vi "connectpython.vi"() -> ()   [LabVIEW 2019]
uses:
  <vilib>/Platform/TimedLoop/XDataNode/timing_clust.ctl
  <vilib>/Platform/TimedLoop/XDataNode/nitl_modes.ctl
  <vilib>/Platform/TimedLoop/XDataNode/wakeup.ctl
  <vilib>/platform/TimedLoop/XDataNode/XDataNode.xnode
  <vilib>/Platform/TimedLoop/XDataNode/XDNodeRunTimeDep.lvlib
panel:
  out "Waveform Chart":dbl(graph)
  out "data out":string
  out "xd":dbl
  out "yd":dbl
  out "phi":dbl
  out "error out":errorcluster
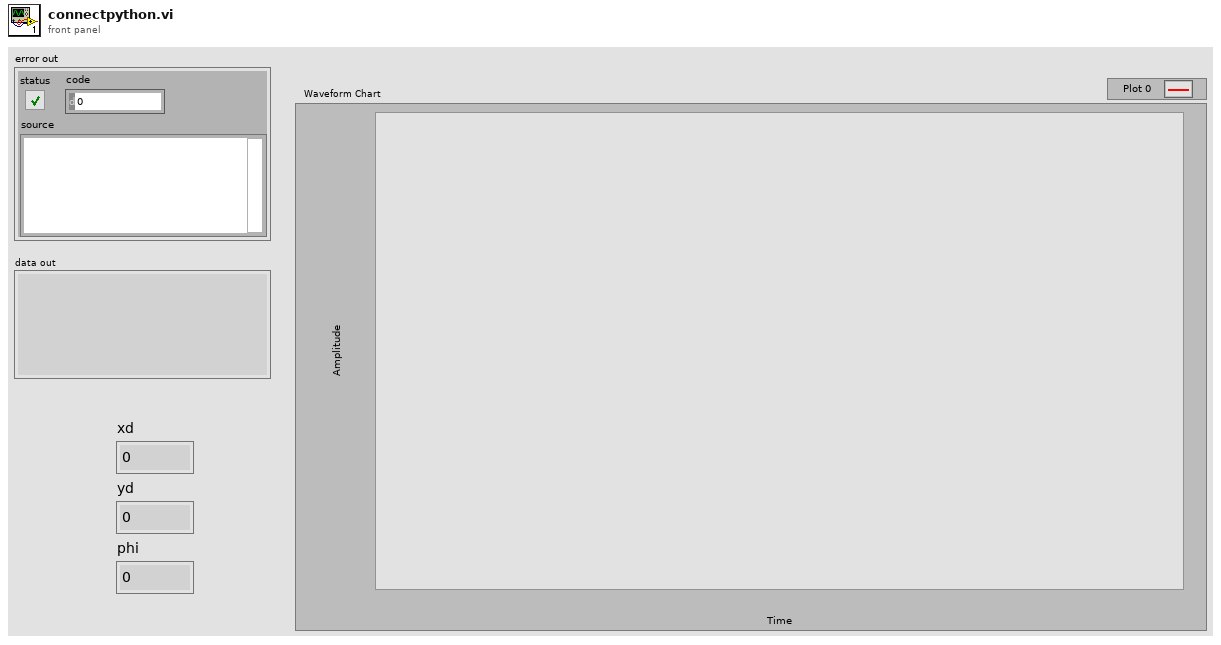
[diagram p1: front panel]
types:
  T1 = typedef "XDNodeRunTimeDep.lvlib/timing_clust.ctl" = cluster{"Expected End [f-1]":u64, "Actual End [f-1]":u64, "Finished Late? [f-1]":bool, "Expected End [i-1]":u64, "Actual End [i-1]":u64, "Finished Late? [i-1]":bool, "Expected Start [i]":u64, "Actual Start [i]":u64, "Expected Start [f]":u64, "Actual Start [f]":u64, "Source Name":string, "Structure Name":string, "Period":i64, "Deadline":i64, "Offset":i64, "Start":i64, "Priority":i32, "Timeout":i32, "Mode":T2, "Wakeup Reason":T3, "Error":errorcluster, "Source Type":string, "Secondary Source Type":string, "Global End Time":u64, "Global Start Time":u64, "Frame Duration":u64, "Iteration Duration":u64, "Assigned CPU":i32, "I/O Scan Engine Mode":u32}
  T2 = typedef "XDNodeRunTimeDep.lvlib/nitl_modes.ctl" = enum32{"No Change", "Process missed periods, maintain original phase", "Discard missed periods, maintain original phase", "Process missed periods, ignore original phase", "Discard missed periods, ignore original phase"}
  T3 = typedef "XDNodeRunTimeDep.lvlib/wakeup.ctl" = enum32{"Normal", "Aborted", "Asynchronous wakeup", "Timing source error", "Timed loop error", "Timeout"}
  T4 = enum16{"Standard", "Buffered", "CRLF", "Immediate"}
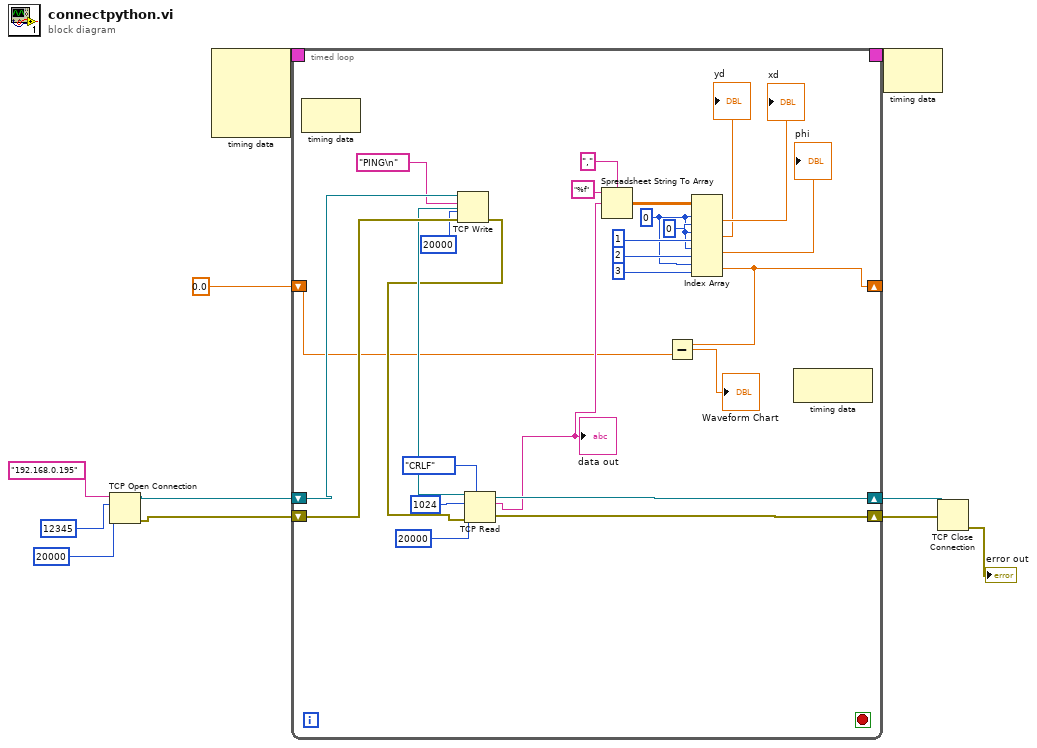
[diagram p0: block diagram]
diagram:
  n1 = TCP Open Connection(address="192.168.0.195", remote port or service name=u16 12345, timeout ms (60000)=20000) -> (connection ID=w5:refnum<k5>, error out=w4:errorcluster)  [unwired: 2 in]
  n2 = node-c288() -> (w11:T1)  [unwired: 4 in]
  n3 = timed-loop {
    timing: w11 -> [_]
    timing-out: [_] -> w10
    shift-right: [w16] -> w8
    shift-left: w4 -> [w22]
    shift-right: [w37] -> w7
    shift-left: w5 -> [w23]
    shift-right: [w14] -> _
    shift-left: 0.0 -> [w13]
    stop <- _ stop-if-true
    w25 = 0 ("index (row)")
    n4 = node-c288() -> ()  [unwired: 1 in, 1 out]
    n5 = TCP Write(connection ID=w23, data in="PING\n", error in (no error)=w22, 9:20000 ("timeout ms (25000)")) -> (connection ID out=w21:refnum<k5>, error out=w20:errorcluster)  [unwired: 1 out]
    n6 = TCP Read(connection ID=w21, bytes to read=1024, error in (no error)=w20, 7:T4."CRLF" ("mode (standard)"), 9:20000 ("timeout ms (25000)")) -> (connection ID out=w37:refnum<k5>, data out=w15:string, error out=w16:errorcluster)
    "data out" <- w15
    n7 = Spreadsheet String To Array(delimiter (Tab)=",", format string="%f", spreadsheet string=w15) -> (array=w33:dbl[][])  [unwired: 1 in]
    n8 = Index Array(array=w33, index (row) #1=w25, index (col) #1=0 ("disabled index (col)"), index (row) #2=w25, index (col) #2=1 ("disabled index (col)"), index (row) #3=w25, index (col) #3=2 ("disabled index (col)"), index (row) #4=w25, index (col) #4=3 ("disabled index (col)")) -> (element #1=→"xd":dbl, element #2=→"yd":dbl, element #3=→"phi":dbl, element #4=w14:dbl)
    n9 = Subtract(x=w14, y=w13) -> (x-y=→"Waveform Chart":dbl)
    n10 = node-c288() -> ()  [unwired: 1 in, 1 out]
  }
  n11 = node-c288(w10) -> ()  [unwired: 1 out]
  n12 = TCP Close Connection(connection ID=w7, error in (no error)=w8) -> (error out=→"error out":errorcluster)  [unwired: 1 in, 1 out]
